vi "Forward Pass (LSTM) 2.vi"(0 "x[t]":T1=[[0.0], [1.0], [0.0]], 2 "c[t-1]":T1=[[0.5], [0.5]] format="%.2f", 4 "h[t-1]":T1=[[0.3], [0.7]] format="%.2f", 5 "param clusters":T2 {"output weights"."Wx[N,M]" format="%.2g"; "output weights"."Wh[M,M]" format="%.2g"; "output weights"."Wc[M,M]" format="%.2g"; "output weights"."bias" format="%.2g"; "candidate weights"."Wx[N,M]" format="%.2g"; "candidate weights"."Wh[M,M]" format="%.2g"; "candidate weights"."bias" format="%.2g"; "forget weights"."Wx[N,M]" format="%.2g"; "forget weights"."Wh[M,M]" format="%.2g"; "forget weights"."Wc[M,M]" format="%.2g"; "forget weights"."bias" format="%.2g"; "input weights"."Wx[N,M]" format="%.2g"; "input weights"."Wh[M,M]" format="%.2g"; "input weights"."Wc[M,M]" format="%.2g"; "input weights"."bias" format="%.2g"}) -> (16 "c[t]":T1=[[-0.7507685227622697], [0.30991943555215495]] format="%.2f", 18 "h[t]":T1=[[-0.5890897103368565], [0.255472245018171]] format="%.2f")   [LabVIEW 2014]
uses:
  <vilib>/Analysis/Matrix/Datatypes/RealMatrix.ctl
  <vilib>/Analysis/Matrix/Numeric/Add/Add - RM,RM.vi
  <vilib>/Analysis/Matrix/NI_Matrix.lvlib
panel:
  out "tanh(c[t])":T1=[[-0.635607218378636], [0.3003638028703052]]
  out "o[t]":T1=[[0.9268140658307178], [0.8505427171212172]] format="%.2f"
  out "h_hat[t]":T1=[[-0.9784223061486208], [-0.594130913568714]] format="%.2f"
  out "i[t]":T1=[[0.06882301233946005], [0.6460540166924326]] format="%.2f"
  out "f[t]":T1=[[0.8024960428618152], [0.022061758603552882]] format="%.2f"
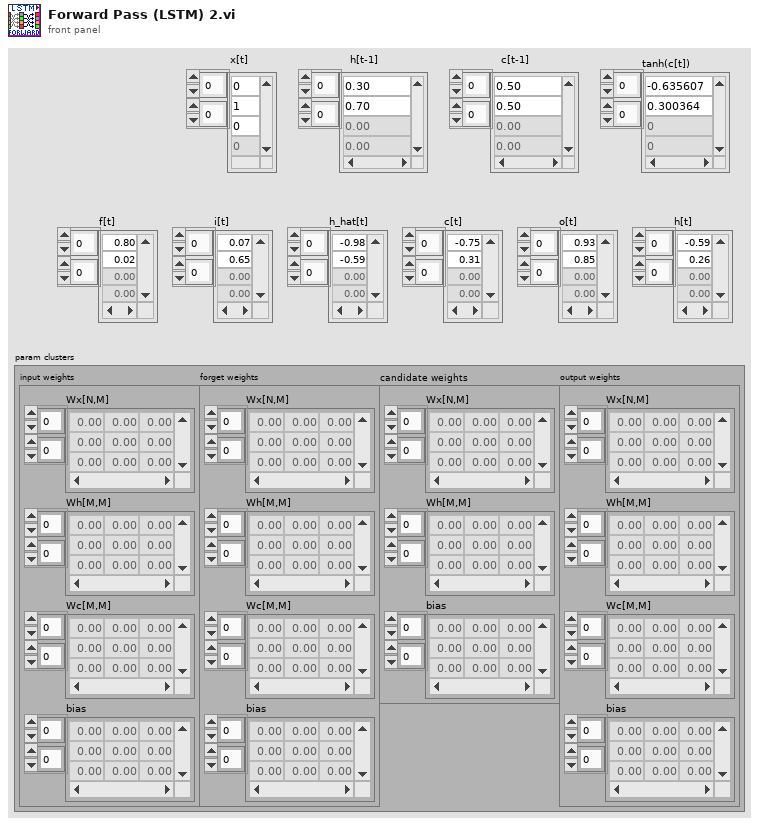
[diagram p1: front panel]
types:
  T1 = typedef "NI_Matrix.lvlib/RealMatrix.ctl" = dbl[][]
  T2 = cluster{"output weights":cluster{"Wx[N,M]":T1, "Wh[M,M]":T1, "Wc[M,M]":T1, "bias":T1}, "candidate weights":cluster{"Wx[N,M]":T1, "Wh[M,M]":T1, "bias":T1}, "forget weights":cluster{"Wx[N,M]":T1, "Wh[M,M]":T1, "Wc[M,M]":T1, "bias":T1}, "input weights":cluster{"Wx[N,M]":T1, "Wh[M,M]":T1, "Wc[M,M]":T1, "bias":T1}}
  T3 = cluster{"Wx[N,M]":T1, "Wh[M,M]":T1, "Wc[M,M]":T1, "bias":T1}
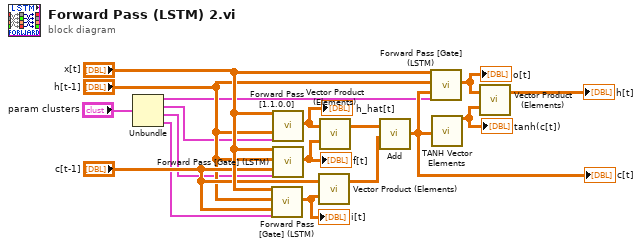
[diagram p0: block diagram]
diagram:
  n1 = Unbundle("param clusters") -> ("output weights"=w4:T3, "candidate weights"=w3:cluster{"Wx[N,M]":T1, "Wh[M,M]":T1, "bias":T1}, "forget weights"=w2:T3, "input weights"=w1:T3)
  n2 = call "Forward Pass [Gate] (LSTM).vi"("x[t]"="x[t]", "h[t-1]"="h[t-1]", "c[t-1]"="c[t-1]", "params"=w1) -> ("Vector"=w10:T1)  [unwired: 15 in]
  "i[t]" <- w10
  n3 = call "Forward Pass [1.1.0.0].vi"("x[t]"="x[t]", "h[t-1]"="h[t-1]", "params"=w3) -> ("Vector"=w12:T1)  [unwired: 16 in]
  "h_hat[t]" <- w12
  n4 = call "Forward Pass [Gate] (LSTM).vi"("x[t]"="x[t]", "h[t-1]"="h[t-1]", "c[t-1]"="c[t-1]", "params"=w2) -> ("Vector"=w11:T1)  [unwired: 15 in]
  "f[t]" <- w11
  n5 = call "Vector Product (Elements).vi"("X"="c[t-1]", "Y"=w10) -> ("X*Y"=w17:T1)  [unwired: 17 in]
  n6 = call "Vector Product (Elements).vi"("X"=w12, "Y"=w11) -> ("X*Y"=w16:T1)  [unwired: 17 in]
  n7 = call-poly <vilib>:"Add.vi"("Real Matrix B"=w17, "Real Matrix A"=w16) -> ("A + B"=w7:T1)
  "c[t]" <- w7
  n8 = call "Forward Pass [Gate] (LSTM).vi"("x[t]"="x[t]", "h[t-1]"="h[t-1]", "c[t-1]"=w7, "params"=w4) -> ("Vector"=w6:T1)  [unwired: 15 in]
  "o[t]" <- w6
  n9 = call "TANH Vector Elements.vi"("X"=w7) -> ("tanh(X)"=w14:T1)  [unwired: 18 in]
  "tanh(c[t])" <- w14
  n10 = call "Vector Product (Elements).vi"("X"=w6, "Y"=w14) -> ("X*Y"=→"h[t]":T1)  [unwired: 17 in]
